vi "CheckVeriStandVersionMatchesLabVIEW.vi"(8 "error in (no error)":errorcluster, 11 "Target (localhost)":refnum<k21>="localhost") -> (0 "error out":errorcluster, 3 "versions match?":bool)   [LabVIEW 2016, in "VeriStandTestUtilities.lvlib"]
uses:
  VeriStandTestUtilities.lvlib
  <vilib>/nisyscfg/Get Installed Components.vi
  <vilib>/nisyscfg/Close (System).vi
  <vilib>/regexp/Match Regular Expression.xnode
  <vilib>/nisyscfg/nisyscfg.lvlib
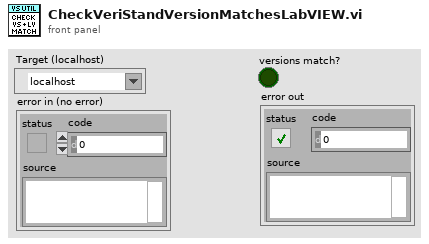
[diagram p1: front panel]
types:
  T1 = typedef "nisyscfg.lvlib/Software 1.2.ctl" = cluster{"title":string, "description":string, "ID":string, "version":string, "component type":T2}
  T2 = typedef "nisyscfg.lvlib/Component Type.ctl" = u32
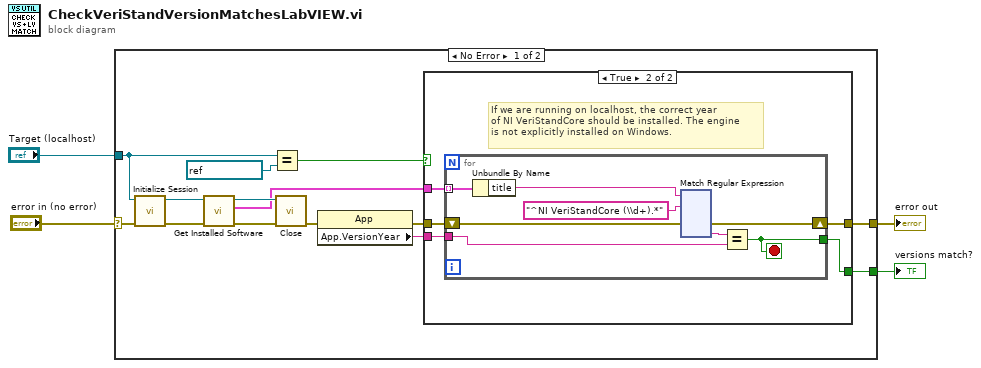
[diagram p0: block diagram]
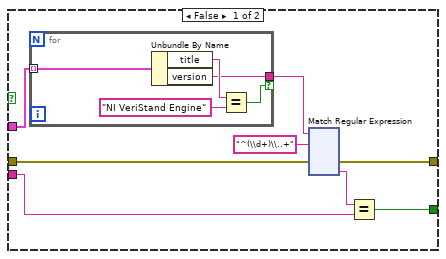
[diagram p2: hidden frame]
diagram:
  n1 = case shown="No Error" "error in (no error)" {
    selector: "error in (no error)" -> [w15 w277]
    tunnel: [w18 _] -> w4
    tunnel: "Target (localhost)" -> [w16 _]
    tunnel: [w14 w277] -> w1
    frame No Error {
      n2 = call <vilib>:"Initialize Session.vi"("error in (no error)"=w15, "Target (localhost)"=w16) -> ("error out"=w10:errorcluster, "Session out"=w13:refnum<k21>)  [unwired: 8 in]
      n3 = call-poly <vilib>:"Get Installed Software.vi"("error in (no error)"=w10, "Session in"=w13) -> ("error out"=w11:errorcluster, "Software Components"=w8:T1[], "Session out"=w12:refnum<k21>)  [unwired: 7 in]
      n4 = Equal?(x=w16, y=refnum<k21> "localhost" ("Target (localhost)")) -> (x = y?=w9:bool)
      n5 = call-poly <vilib>:"Close.vi"("error in (no error)"=w11, "Session in"=w12) -> ("error out"=w6:errorcluster)  [unwired: 9 in]
      n6 = property class="App"(error in=w6) -> (error out=w7:errorcluster, "App.VersionYear"=w5:string)  [unwired: 1 in, 1 out]
      n7 = case shown="True" w9 {
        tunnel: [w23 w150] -> w18
        tunnel: [w19 w148] -> w14
        tunnel: w8 -> [w26 w152]
        tunnel: w7 -> [w20 w149]
        tunnel: w5 -> [w21 w151]
        frame False {
          n8 = for {
            tunnel: w26 -> [w147] mode=indexing
            tunnel: [w144] -> w25 if=w143
            n9 = Unbundle By Name(w147) -> ("title"=w146:string, "version"=w144:string)
            n10 = Equal?(x=w146, y="NI VeriStand Engine") -> (x = y?=w143:bool)
          }
          n11 = xnode "Match Regular Expression"("input string"=w25, "regular expression"="^(\\d+)\\..+" ("y"), "error in"=w20) -> ("error out"=w19:errorcluster, "submatch 1"=w22:string)  [unwired: 3 in, 4 out]
          n12 = Equal?(x=w22, y=w21) -> (x = y?=w23:bool)
        }
        frame True {
          # "If we are running on localhost, the correct year\nof NI VeriStandCore should be installed. The engine\nis not explicitly installed on Windows."
          n13 = for {
            tunnel: w152 -> [w160] mode=indexing
            tunnel: w151 -> [w156]
            tunnel: [w155] -> w150
            shift-right: [w153] -> w148
            shift-left: w149 -> [w154]
            stop <- w155 stop-if-true
            n14 = Unbundle By Name(w160) -> ("title"=w158:string)
            n15 = xnode "Match Regular Expression"("input string"=w158, "regular expression"="^NI VeriStandCore (\\d+).*" ("y"), "error in"=w154) -> ("error out"=w153:errorcluster, "submatch 1"=w157:string)  [unwired: 3 in, 4 out]
            n16 = Equal?(x=w157, y=w156) -> (x = y?=w155:bool)
          }
        }
      }
    }
    frame Error {
    }
  }
  "versions match?" <- w4
  "error out" <- w1
